vi "FOCUS_V42.vi"(9 "X-pixels":sgl=256.0, 11 "Run":bool) -> (0 "Retrace pixels":sgl, 10 "Pixel Clock (Hz)":sgl)   [LabVIEW 2010] (continued)
                      tunnel: w5383 -> [w5401 w5419]
                      tunnel: w5352 -> [w5400 w5418]
                      tunnel: [w5399 w5417] -> w5382
                      tunnel: [w5398 w5416] -> w5381
                      tunnel: [w5398 w5416] -> w5368
                      tunnel: w5367 -> [_ _]
                      tunnel: w5360 -> [w5397 _]
                      tunnel: w5359 -> [w5393 w5414]
                      tunnel: [w5395 w5412] -> w5341
                      tunnel: w5340 -> [w5394 _]
                      frame False {
                        n2972 = case shown="True" w5394 {
                          tunnel: [w5402 w5403] -> w5395
                          tunnel: w5393 -> [w5402 _]
                          frame False {
                          }
                          frame True {
                            n2973 = local read "scattering length [µm]"() -> (w5411:sgl)
                            n2974 = local read "z-step (um)"() -> (w5407:sgl)
                            n2975 = Divide(x=w5407, y=w5411) -> (x/y=w5408:sgl)
                            n2976 = Exponential(1:w5408) -> (0:w5409:sgl)
                            n2977 = local read "Intensity"() -> (w5410:sgl)
                            n2978 = local read "IntensityScaleMax"() -> (w5404:sgl)
                            n2979 = Multiply(x=w5410, y=w5409) -> (x*y=w5405:sgl)
                            n2980 = In Range and Coerce(upper limit=sgl 0.0, x=w5405, lower limit=w5404) -> (coerced(x)=w5403:sgl)  [unwired: 1 out]
                            n2981 = local write "Intensity"(w5403) -> ()
                          }
                        }
                        n2982 = Build Array(w5397, w5395) -> (w5396:dbl[])
                        n2983 = call-poly <vilib>:"DAQmx Write (Analog 1D DBL NChan 1Samp).vi"("task/channels in"=w5401, "data"=w5396, "error in"=w5400) -> ("task out"=w5398:refnum<k21>, "error out"=w5399:errorcluster)  [unwired: 10 in, 1 out]
                      }
                      frame True {
                        n2984 = local read "IntensityScaleMax"() -> (w5413:sgl)
                        n2985 = In Range and Coerce(upper limit=sgl 0.0, x=w5414, lower limit=w5413) -> (coerced(x)=w5412:sgl)  [unwired: 1 out]
                        n2986 = local write "Intensity"(w5412) -> ()
                        n2987 = Build Array(0.0 ("data"), w5412) -> (w5421:dbl[])
                        n2988 = call-poly <vilib>:"DAQmx Write (Analog 1D DBL NChan 1Samp).vi"("task/channels in"=w5419, "data"=w5421, "error in"=w5418) -> ("task out"=w5416:refnum<k21>, "error out"=w5417:errorcluster)  [unwired: 10 in, 1 out]
                      }
                    }
                    n2989 = case shown="False" w5326 {
                      tunnel: [w5431 w5457] -> w5371
                      tunnel: [w5430 w5456] -> w5370
                      tunnel: [w5428 w5454] -> w5356
                      tunnel: w5369 -> [w5427 w5457]
                      tunnel: w5368 -> [w5426 _]
                      tunnel: w5367 -> [w5425 w5456]
                      tunnel: w5358 -> [w5424 w5455]
                      tunnel: [w5423 w5455] -> w5357
                      tunnel: w5362 -> [w5422 w5454]
                      frame False {
                        n2990 = flat-sequence {
                          tunnel: sgl 100.0 ("Time interval [s]") -> [w5443]
                          tunnel: [w5443] -> w5437
                          tunnel: [w5439] -> w5436
                          tunnel: [w5438] -> w5435
                          tunnel: w5427 -> [w5441]
                          tunnel: w5425 -> [w5440]
                          tunnel: [w5450] -> w5434
                          tunnel: [w5449] -> w5433
                          tunnel: [w5448] -> w5432
                          tunnel: w5437 -> [w5450]
                          tunnel: w5436 -> [w5449]
                          tunnel: w5435 -> [w5448]
                          tunnel: w5424 -> [w5447]
                          tunnel: w5422 -> [w5446]
                          tunnel: [w5445] -> w5428
                          tunnel: [w5444] -> w5423
                          tunnel: [w5453] -> w5431
                          tunnel: w5434 -> [w5452]
                          tunnel: w5433 -> [w5453]
                          tunnel: w5432 -> [w5451]
                          tunnel: [w5451] -> w5430
                          tunnel: w5426 -> [_]
                          frame #0 {
                            w5442 = FALSE ("data")
                            n2991 = local write "Shutter open"(w5442) -> ()
                            n2992 = call-poly <vilib>:"DAQmx Write (Digital Bool 1Line 1Point).vi"("task/channels in"=w5441, "data"=w5442, "error in"=w5440) -> ("task out"=w5439:refnum<k21>, "error out"=w5438:errorcluster)  [unwired: 10 in, 1 out]
                          }
                          frame #1 {
                            n2993 = call <vilib>:"DAQmx Stop Task.vi"("task/channels in"=w5447, "error in"=w5446) -> ("task out"=w5444:refnum<k21>, "error out"=w5445:errorcluster)  [unwired: 12 in]
                          }
                          frame #2 {
                            n2994 = Wait (ms)(milliseconds to wait=w5452) -> ()  [unwired: 1 out]
                          }
                        }
                      }
                      frame True {
                      }
                    }
                    n2995 = call "ConvertImagesDataFOCUS.vi"("Save mode"=w5320, "Image3"=w5324, "Image2"=w5333, "Image1"=w5334) -> ("Data"=w5332:u8[])
                    n2996 = Set File Position(refnum=w5338, from (0:start)=enum16{"start", "end", "current"}."current" ("pos mode (0:2)"), error in=w5337) -> (refnum out=w5319:refnum<file>, error out=w5318:errorcluster)  [unwired: 1 in]
                    n2997 = Write to Binary File(file (use dialog)=w5319, data=w5332, error in=w5318, 5:FALSE ("prepend array or string size? (T)")) -> (refnum out=w5336:refnum<file>, error out=w5335:errorcluster)  [unwired: 2 in, 1 out]
                    n2998 = local read "Y-lines"() -> (w5380:sgl)
                    n2999 = Multiply(x=w5353, y=w5380) -> (x*y=w5378:sgl)
                    n3000 = Replace Array Subset(array=w5385, new element=w5334, index (row)=0 ("disabled index (row)"), index (col)=w5378) -> (w5384:u8[][])
                    n3001 = Replace Array Subset(array=w5387, new element=w5333, index (row)=0 ("disabled index (row)"), index (col)=w5378) -> (w5386:u8[][])
                  }
                  n3002 = Not Equal?(x=w5253, y=w5254) -> (x != y?=w5255:bool)
                  n3003 = local write "IntDevUsed"(w5255) -> ()
                  n3004 = Close File(refnum=w5240, error in=w5239) -> ()  [unwired: 2 out]
                  n3005 = flat-sequence {
                    tunnel: [w5302] -> w5264
                    tunnel: w5266 -> [w5302]
                    tunnel: w5265 -> [w5301]
                    tunnel: [w5301] -> w5263
                    frame #0 {
                      n3006 = Tick Count (ms)() -> (millisecond timer value=w5303:u32)
                      n3007 = local write "stop"(w5303) -> ()
                    }
                  }
                }
                frame 5 {
                  w5744 = sgl 1000000.0 ("y")
                  w5776 = 0.0 ("X Scale.Range:Minimum")
                  w5783 = TRUE ("Visible")
                  # "User-defined line 3D"
                  n3008 = Greater Or Equal?(x=w5710, y=u16 3) -> (x >= y?=w5708:bool)
                  n3009 = property on="Property Node" class="VI"() -> ("VI Path"=w5738:path)  [unwired: 2 in, 2 out]
                  n3010 = property on="Property Node" class="VI"() -> ("VI Path"=w5719:path)  [unwired: 2 in, 2 out]
                  n3011 = flat-sequence {
                    tunnel: w5785 -> [w5800]
                    tunnel: [w5800] -> w5784
                    frame #0 {
                      n3012 = Tick Count (ms)() -> (millisecond timer value=w5801:u32)
                      n3013 = local write "start"(w5801) -> ()
                    }
                  }
                  n3014 = Unbundle By Name(w5723) -> ("status"=w5757:bool)
                  n3015 = Increment(x=w5734) -> (x+1=w5733:sgl)
                  n3016 = Tick Count (ms)() -> (millisecond timer value=w5789:u32)
                  n3017 = Strip Path(path=w5738) -> (stripped path=w5737:path)  [unwired: 1 out]
                  n3018 = Strip Path(path=w5719) -> (stripped path=w5718:path)  [unwired: 1 out]
                  n3019 = local read "X-pixels FreeLine"() -> (w5743:sgl)
                  n3020 = local read "Y-lines FreeLine"() -> (w5745:sgl)
                  n3021 = Build Path(base path=w5737, name or relative path="FreeLine.tmp") -> (appended path=w5736:path)
                  n3022 = Build Path(base path=w5718, name or relative path="EEG.tmp") -> (appended path=w5717:path)
                  n3023 = call <vilib>:"Open_Create_Replace File.vi"("advisory dialog? (display:T)"=FALSE, "function (open:0)"=T8."create or replace", "file path"=w5736) -> ("error out"=w5727:errorcluster, "refnum"=w5729:refnum<file>)  [unwired: 5 in, 2 out]
                  n3024 = Unbundle By Name(w5759) -> ("status"=w5758:bool)
                  n3025 = call <vilib>:"Open_Create_Replace File.vi"("advisory dialog? (display:T)"=FALSE, "function (open:0)"=T8."create or replace", "file path"=w5717) -> ("error out"=w5715:errorcluster, "refnum"=w5714:refnum<file>)  [unwired: 5 in, 2 out]
                  n3026 = Divide(x=w5744, y=w5743) -> (x/y=w5742:sgl)
                  n3027 = Multiply(x=w5745, y=w5743) -> (x*y=w5746:sgl)
                  n3028 = local read "XScale"() -> (w5777:bool)
                  n3029 = Greater?(x=w5746, y=w5744) -> (0:w5747:bool)
                  n3030 = Select(t=w5742, s=w5747, f=w5745) -> (s? t:f=w5741:sgl)
                  n3031 = case shown="True" w5777 {
                    tunnel: [w5796 w5797] -> w5775
                    tunnel: w5741 -> [w5796 _]
                    tunnel: w5743 -> [_ w5797]
                    frame False {
                    }
                    frame True {
                    }
                  }
                  n3032 = Set File Position(refnum=w5729, from (0:start)=enum16{"start", "end", "current"}."start" ("pos mode (rel. to end:1)"), error in=w5727) -> (refnum out=w5707:refnum<file>, error out=w5706:errorcluster)  [unwired: 1 in]
                  n3033 = Write to Binary File(file (use dialog)=w5707, data=w5730, error in=w5706, 5:FALSE ("prepend array or string size? (T)")) -> (refnum out=w5728:refnum<file>, error out=w5726:errorcluster)  [unwired: 2 in, 1 out]
                  n3034 = while {
                    tunnel: [w5841] -> w5790
                    tunnel: [w5839] -> w5787
                    tunnel: w5791 -> [w5870]
                    tunnel: w5784 -> [w5863]
                    shift-right: [w5846] -> w5751
                    shift-left: w5792 -> [w5902]
                    tunnel: w5748 -> [w5817]
                    shift-right: [w5848] -> w5752
                    shift-left: w5792 -> [w5901]
                    shift-right: [w5896] -> _
                    shift-left: w5789 -> [w5897]
                    tunnel: w5781 -> [w5873]
                    tunnel: w5780 -> [w5864]
                    tunnel: [w5872] -> w5778
                    tunnel: [w5871] -> w5779
                    shift-right: [w5876] -> w5732
                    shift-left: w5774 -> [w5878]
                    tunnel: w5764 -> [w5874]
                    tunnel: w5763 -> [w5862]
                    tunnel: [w5874] -> w5761
                    tunnel: [w5862] -> w5762
                    tunnel: [w5866] -> w5760
                    tunnel: w5758 -> [w5861]
                    tunnel: w5757 -> [w5857]
                    shift-right: [w5850] -> w5749
                    shift-left: w5728 -> [w5852]
                    shift-right: [w5849] -> w5750
                    shift-left: w5726 -> [w5851]
                    tunnel: w5733 -> [w5843]
                    tunnel: w5725 -> [w5837]
                    tunnel: w5723 -> [w5836]
                    tunnel: [w5835] -> w5724
                    tunnel: [w5834] -> w5722
                    shift-right: [w5826] -> w5713
                    shift-left: w5714 -> [w5828]
                    shift-right: [w5825] -> w5712
                    shift-left: w5715 -> [w5827]
                    tunnel: w5711 -> [w5823]
                    tunnel: w5710 -> [w5813]
                    tunnel: w5708 -> [w5808]
                    i -> [w5844]
                    stop <- w5853 stop-if-true
                    # "DIO Read reads one\nline of data at a time"
                    n3035 = Unbundle By Name(w5862) -> ("status"=w5860:bool)
                    n3036 = Unbundle By Name(w5864) -> ("status"=w5859:bool)
                    n3037 = Equal To 0?(x=w5844) -> (x = 0?=w5883:bool)
                    n3038 = Unbundle By Name(w5863) -> ("status"=w5858:bool)
                    n3039 = local read "End experiment"() -> (w5855:bool)
                    n3040 = local read "Y-lines FreeLine"() -> (w5865:sgl)
                    n3041 = case shown="False" w5883 {
                      tunnel: w5817 -> [w5962 w5965]
                      tunnel: [w5962 w5964] -> w5816
                      tunnel: w5823 -> [_ w5963]
                      tunnel: [sgl 0.0 w5963] -> w5818
                      frame False {
                      }
                      frame True {
                        n3042 = Add(x=w5965, y=w5963) -> (x+y=w5964:sgl)
                      }
                    }
                    n3043 = call-poly <vilib>:"DAQmx Read (Analog 2D DBL NChan NSamp).vi"("task/channels in"=w5873, "number of samples per channel"=w5816, "error in"=w5864) -> ("task out"=w5872:refnum<k21>, "data"=w5820:dbl[][], "error out"=w5871:errorcluster)  [unwired: 10 in]
                    n3044 = Array Subset(array=w5820, index (col)=w5818) -> (w5819:dbl[][])  [unwired: 3 in]
                    n3045 = local read "stop 2"() -> (w5856:bool)
                    n3046 = Transpose 2D Array(2D array=w5819) -> (transposed array=w5830:dbl[][])
                    n3047 = Increment(x=w5844) -> (x+1=w5875:i32)
                    n3048 = call-poly <vilib>:"DAQmx Read (Digital 1D U32 1Chan NSamp).vi"("task/channels in"=w5870, "number of samples per channel"=w5816, "error in"=w5863) -> ("task out"=w5842:refnum<k21>, "data"=w5822:u32[], "error out"=w5840:errorcluster)  [unwired: 10 in]
                    n3049 = Build Array (concatenate)(w5878, w5830) -> (w5877:dbl[][])
                    n3050 = Multiply(x="z frequency", y=w5817) -> (x*y=w5833:dbl)
                    n3051 = Index Array(array=w5830, index (col)=0 ("disabled index (col)")) -> (element=w5880:dbl[])  [unwired: 1 in]
                    n3052 = Equal?(x=w5875, y=w5865) -> (x = y?=w5854:bool)
                    n3053 = local write "#"(w5875) -> ()
                    n3054 = Index Array(array=w5830, index (col)=1 ("disabled index (col)")) -> (element=w5879:dbl[])  [unwired: 1 in]
                    n3055 = Array Subset "Extract DI0"(array=w5822, index=w5818) -> (w5821:u32[])  [unwired: 1 in]
                    n3056 = Index Array(array=w5830, index (col)=3 ("disabled index (col)")) -> (element=w5824:dbl[])  [unwired: 1 in]
                    n3057 = local read "Overlay Images"() -> (w5884:bool)
                    n3058 = property class="DAQmx Timing"(reference=w5837, error in=w5836, "Sample Clock:Rate"=w5833) -> (reference out=w5835:refnum<k21>, error out=w5834:errorcluster)
                    n3059 = Compound Arithmetic op=OR(w5854, w5855, w5856, w5857, w5858, w5859, w5860, w5861) -> (w5853:bool)
                    n3060 = Array Subset(array=w5877, index (row)=w5817) -> (w5876:dbl[][])  [unwired: 3 in]
                    n3061 = local read "x scale"() -> (w5890:dbl)
                    n3062 = local read "y scale"() -> (w5888:dbl)
                    n3063 = Split Number(x=w5821) -> (hi(x)=w5815:u16[], lo(x)=w5814:u16[])
                    n3064 = property class="DAQmx Read"(reference=w5842, error in=w5840) -> (reference out=w5841:refnum<k21>, error out=w5839:errorcluster, "Status:Available Samples Per Channel"=→"Scan Backlock":u32)
                    n3065 = case shown="0, Default" w5813 {
                      tunnel: w5815 -> [w5914 w5919 w5924 w5929 w5934 w5939]
                      tunnel: [w5913 w5918 w5921 w5928 w5933 w5936] -> w5812
                      tunnel: [w5911 w5916 w5923 w5926 w5931 w5938] -> w5811
                      tunnel: w5814 -> [w5912 w5917 w5922 w5927 w5932 w5937]
                      tunnel: [w5910 w5915 w5920 w5925 w5930 w5935] -> w5810
                      frame 0, Default {
                        n3066 = Split Number(x=w5914) -> (hi(x)=w5913:u8[], lo(x)=w5911:u8[])
                        n3067 = Split Number(x=w5912) -> (lo(x)=w5910:u8[])  [unwired: 1 out]
                      }
                      frame 1 {
                        n3068 = Split Number(x=w5919) -> (hi(x)=w5918:u8[], lo(x)=w5915:u8[])
                        n3069 = Split Number(x=w5917) -> (lo(x)=w5916:u8[])  [unwired: 1 out]
                      }
                      frame 2 {
                        n3070 = Split Number(x=w5924) -> (hi(x)=w5920:u8[], lo(x)=w5923:u8[])
                        n3071 = Split Number(x=w5922) -> (lo(x)=w5921:u8[])  [unwired: 1 out]
                      }
                      frame 3 {
                        n3072 = Split Number(x=w5929) -> (hi(x)=w5928:u8[], lo(x)=w5926:u8[])
                        n3073 = Split Number(x=w5927) -> (lo(x)=w5925:u8[])  [unwired: 1 out]
                      }
                      frame 4 {
                        n3074 = Split Number(x=w5934) -> (hi(x)=w5933:u8[], lo(x)=w5930:u8[])
                        n3075 = Split Number(x=w5932) -> (lo(x)=w5931:u8[])  [unwired: 1 out]
                      }
                      frame 5 {
                        n3076 = Split Number(x=w5939) -> (hi(x)=w5935:u8[], lo(x)=w5938:u8[])
                        n3077 = Split Number(x=w5937) -> (lo(x)=w5936:u8[])  [unwired: 1 out]
                      }
                    }
                    n3078 = Tick Count (ms)() -> (millisecond timer value=w5898:u32)
                    n3079 = Multiply(x=w5879, y=w5888) -> (x*y=w5892:dbl[])
                    n3080 = Multiply(x=w5890, y=w5880) -> (x*y=w5894:dbl[])
                    n3081 = local read "x offset"() -> (w5889:dbl)
                    n3082 = case shown="True" w5884 {
                      tunnel: w5812 -> [w5967 w5970]
                      tunnel: [w5967 w5968] -> w5886
                      tunnel: w5811 -> [w5966 w5969]
                      tunnel: [w5966 _] -> w5885
                      frame False {
                      }
                      frame True {
                        n3083 = To Word Integer(number=w5970) -> (16bit integer=w5975:i16[])
                        n3084 = Subtract(x=w5975, y=w5969) -> (x-y=w5976:i16[])
                        n3085 = Add(x=w5975, y=w5969) -> (x+y=w5980:i16[])
                        n3086 = Increment(x=w5980) -> (x+1=w5971:i16[])
                        n3087 = Divide(x=w5976, y=w5971) -> (x/y=w5972:dbl[])
                        n3088 = Absolute Value(x=w5976) -> (abs(x)=w5978:i16[])
                        n3089 = Multiply(x=w5972, y=u8 2) -> (x*y=w5974:dbl[])
                        n3090 = Round To Nearest(number=w5974) -> (nearest integer value=w5987:dbl[])
                        n3091 = Divide(x=w5978, y=2.0) -> (x/y=w5981:dbl[])
                        n3092 = Divide(x=w5980, y=2.0) -> (x/y=w5982:dbl[])
                        n3093 = Add(x=w5981, y=w5982) -> (x+y=w5984:dbl[])
                        n3094 = Divide(x=w5984, y=5.0) -> (x/y=w5985:dbl[])
                        n3095 = Round To Nearest(number=w5985) -> (nearest integer value=w5986:dbl[])
                        n3096 = Multiply(x=5.0 ("y"), y=w5986) -> (x*y=w5988:dbl[])
                        n3097 = Add(x=w5987, y=w5988) -> (x+y=w5989:dbl[])
                        n3098 = Subtract(x=w5989, y=2.0) -> (x-y=w5992:dbl[])
                        n3099 = To Unsigned Byte Integer(number=w5992) -> (unsigned 8bit integer=w5968:u8[])
                      }
                    }
                    n3100 = Subtract(x=w5898, y=w5897) -> (x-y=w5899:u32)
                    n3101 = local read "y offset"() -> (w5887:dbl)
                    n3102 = local read "Image Update [ms]"() -> (w5869:u32)
                    n3103 = Add(x=w5892, y=w5887) -> (x+y=w5891:dbl[])
                    n3104 = Add(x=w5889, y=w5894) -> (x+y=w5893:dbl[])
                    n3105 = Subtract(x=w5844, y=w5817) -> (x-y=w5866:sgl)
                    n3106 = case shown="True" w5808 {
                      tunnel: w5812 -> [w5906 w5909]
                      tunnel: w5811 -> [w5903 w5908]
                      tunnel: w5810 -> [w5905 _]
                      tunnel: [w5904 w5907] -> w5809
                      frame True {
                        n3107 = Interleave 1D Arrays(w5903, w5906, w5905) -> (w5904:u8[])
                      }
                      frame False {
                        n3108 = Interleave 1D Arrays(w5909, w5908) -> (w5907:u8[])
                      }
                    }
                    n3109 = Multiply(x=w5869, y=u32 20) -> (x*y=w5867:u32)
                    n3110 = Greater Or Equal?(x=w5899, y=w5867) -> (x >= y?=w5900:bool)
                    n3111 = Greater Or Equal?(x=w5844, y=w5843) -> (x >= y?=w5845:bool)
                    n3112 = case shown="True" w5845 {
                      tunnel: w5902 -> [w5946 w5959]
                      tunnel: w5901 -> [w5945 w5953]
                      tunnel: w5886 -> [w5944 w5957]
                      tunnel: w5885 -> [w5943 w5950]
                      tunnel: [w5942 w5947] -> w5848
                      tunnel: [w5941 w5960] -> w5846
                      tunnel: w5844 -> [w5940 _]
                      frame False {
                        n3113 = Replace Array Subset(array=w5946, new element=w5944, index (col)=w5940) -> (w5941:u8[][])  [unwired: 1 in]
                        n3114 = Replace Array Subset(array=w5945, new element=w5943, index (col)=w5940) -> (w5942:u8[][])  [unwired: 1 in]
                      }
                      frame True {
                        n3115 = Transpose 2D Array(2D array=w5953) -> (transposed array=w5951:u8[][])
                        n3116 = Transpose 2D Array(2D array=w5959) -> (transposed array=w5958:u8[][])
                        n3117 = Build Array (concatenate)(w5951, w5950) -> (w5952:u8[][])
                        n3118 = Build Array (concatenate)(w5958, w5957) -> (w5956:u8[][])
                        n3119 = Transpose 2D Array(2D array=w5952) -> (transposed array=w5948:u8[][])
                        n3120 = Transpose 2D Array(2D array=w5956) -> (transposed array=w5955:u8[][])
                        n3121 = Array Subset(array=w5955, index (col)=1 ("index")) -> (w5960:u8[][])  [unwired: 3 in]
                        n3122 = Array Subset(array=w5948, index (col)=1 ("index")) -> (w5947:u8[][])  [unwired: 3 in]
                      }
                    }
                    n3123 = Set File Position(refnum=w5828, from (0:start)=enum16{"start", "end", "current"}."current" ("pos mode (0:2)"), error in=w5827) -> (refnum out=w5807:refnum<file>, error out=w5806:errorcluster)  [unwired: 1 in]
                    n3124 = Write to Binary File(file (use dialog)=w5807, data=w5824, error in=w5806, 5:FALSE ("prepend array or string size? (T)")) -> (refnum out=w5826:refnum<file>, error out=w5825:errorcluster)  [unwired: 2 in, 1 out]
                    n3125 = Set File Position(refnum=w5852, from (0:start)=enum16{"start", "end", "current"}."current" ("pos mode (0:2)"), error in=w5851) -> (refnum out=w5804:refnum<file>, error out=w5803:errorcluster)  [unwired: 1 in]
                    n3126 = Write to Binary File(file (use dialog)=w5804, data=w5809, error in=w5803, 5:FALSE ("prepend array or string size? (T)")) -> (refnum out=w5850:refnum<file>, error out=w5849:errorcluster)  [unwired: 2 in, 1 out]
                    n3127 = Bundle(w5893, w5891) -> (w5895:cluster{dbl[], dbl[]})  [unwired: 1 in]
                    n3128 = case shown="True" w5900 {
                      tunnel: [w5993 w5997] -> w5896
                      tunnel: w5897 -> [w5993 _]
                      tunnel: w5895 -> [_ w5996]
                      tunnel: w5846 -> [_ w5995]
                      tunnel: w5848 -> [_ w5994]
                      frame False {
                      }
                      frame True {
                        n3129 = local write "XY Graph 3"(w5996) -> ()
                        n3130 = local write "XY Graph 4"(w5996) -> ()
                        n3131 = local write "Image 4"(w5994) -> ()
                        n3132 = local write "Image 3"(w5995) -> ()
                        n3133 = Tick Count (ms)() -> (millisecond timer value=w5997:u32)
                      }
                    }
                  }
                  n3134 = property on="Image 2" class="IntGraph (strict)"() -> ("Color Table"=w5782:u32[])  [unwired: 2 in, 2 out]
                  n3135 = property on="Image 3" class="IntGraph (strict)"("X Scale.Range:Minimum"=w5776, "X Scale.Range:Maximum"=w5775, "Y Scale.Range:Minimum"=w5776, "Y Scale.Range:Maximum"=w5741, "Visible"=w5783, "Color Table"=w5782) -> ()  [unwired: 2 in, 2 out]
                  n3136 = property on="Image 4" class="IntGraph (strict)"("X Scale.Range:Minimum"=w5776, "X Scale.Range:Maximum"=w5775, "Y Scale.Range:Minimum"=w5776, "Y Scale.Range:Maximum"=w5741, "Visible"=w5783, "Color Table"=w5782) -> ()  [unwired: 2 in, 2 out]
                  n3137 = property on="Histogram1" class="XYGraph (strict)"("X Scale.Range:Minimum"=w5776, "X Scale.Range:Maximum"=w5775) -> ()  [unwired: 2 in, 2 out]
                  n3138 = property on="Histogram2" class="XYGraph (strict)"("X Scale.Range:Minimum"=w5776, "X Scale.Range:Maximum"=w5775) -> ()  [unwired: 2 in, 2 out]
                  n3139 = Close File(refnum=w5749, error in=w5750) -> ()  [unwired: 2 out]
                  n3140 = Close File(refnum=w5713, error in=w5712) -> ()  [unwired: 2 out]
                  n3141 = Array Subset(array=w5732, index (col)=0 ("index"), length (col)=3 ("length")) -> (w5765:dbl[][])  [unwired: 2 in]
                  n3142 = Index Array(array=w5765, index (col)=0 ("disabled index (col)")) -> (element=w5772:dbl[])  [unwired: 1 in]
                  n3143 = flat-sequence {
                    tunnel: w5787 -> [w5798]
                    tunnel: [w5798] -> w5786
                    frame #0 {
                      n3144 = Tick Count (ms)() -> (millisecond timer value=w5799:u32)
                      n3145 = local write "stop"(w5799) -> ()
                    }
                  }
                  n3146 = Array Size(array=w5772) -> (size(s)=w5771:i32)
                  n3147 = Multiply(x=w5771, y=3) -> (x*y=w5769:i32)
                  n3148 = Reshape Array(w5765, w5769) -> (w5768:dbl[])
                  n3149 = local write "Positions"(w5768) -> ()
                }
              }
            }
            frame True {
              n3150 = local read "scans to read"() -> (w6007:sgl)
              n3151 = local read "Number of Frames"() -> (w6004:sgl)
              n3152 = Multiply(x=w6007, y=w6006) -> (x*y=w6003:sgl)
              n3153 = Multiply(x=w6005, y=w6004) -> (x*y=w6010:sgl)
              n3154 = Reciprocal(x=w6003) -> (1/x=w6002:sgl)
              n3155 = local write "Frame rate [Hz]"(w6002) -> ()
              n3156 = case shown="0, Default" w6050 {
                tunnel: w6049 -> [w6084 w6319 w6507]
                tunnel: w6048 -> [w6085 w6320 w6508]
                tunnel: w6047 -> [w6073 w6308 w6496]
                tunnel: w6046 -> [w6083 w6318 w6506]
                tunnel: w6045 -> [w6072 w6307 w6495]
                tunnel: w6044 -> [w6078 w6313 w6501]
                tunnel: w6043 -> [w6077 w6312 w6500]
                tunnel: w6042 -> [w6082 w6317 w6505]
                tunnel: w6041 -> [w6081 w6316 w6504]
                tunnel: w6040 -> [w6087 w6298 w6486]
                tunnel: w6039 -> [w6068 w6297 w6485]
                tunnel: w6038 -> [w6088 w6322 w6510]
                tunnel: w6037 -> [w6069 w6304 w6492]
                tunnel: w6036 -> [w6089 w6323 w6511]
                tunnel: [w6089 w6323 w6511] -> w6035
                tunnel: [w6069 w6304 w6492] -> w6033
                tunnel: [w6088 w6322 w6510] -> w6034
                tunnel: [w6068 w6295 w6483] -> w6031
                tunnel: [w6087 w6296 w6484] -> w6032
                tunnel: [768 ("DataOffset") 768 ("DataOffset") 768 ("DataOffset")] -> w6030
                tunnel: [0 ("DataOffset") 0 ("DataOffset") 0 ("DataOffset")] -> w6029
                tunnel: [0 ("DataOffset") 0 ("DataOffset") 0 ("DataOffset")] -> w6028
                tunnel: [w6079 w6314 w6502] -> w6027
                tunnel: [w6080 w6315 w6503] -> w6026
                tunnel: [w6075 w6310 w6498] -> w6025
                tunnel: [w6076 w6311 w6499] -> w6024
                tunnel: [w6073 w6308 w6496] -> w6023
                tunnel: [w6085 w6320 w6508] -> w6022
                tunnel: [w6084 w6319 w6507] -> w6021
                tunnel: [w6072 w6307 w6495] -> w6020
                tunnel: [w6083 w6318 w6506] -> w6019
                tunnel: w6018 -> [w6055 w6283 w6497]
                tunnel: w6017 -> [w6062 w6301 w6489]
                tunnel: w6007 -> [_ w6290 w6482]
                tunnel: w6016 -> [w6061 w6289 w6481]
                tunnel: w6015 -> [w6060 w6288 w6480]
                tunnel: w6014 -> [w6059 w6286 w6478]
                tunnel: w6013 -> [w6058 w6287 w6479]
                tunnel: [w6057 w6286 w6478] -> w6012
                tunnel: [w6056 w6287 w6479] -> w6011
                tunnel: w6010 -> [_ w6285 _]
                tunnel: w6009 -> [_ w6284 _]
                tunnel: [_ w6281 w6473] -> w6008
                tunnel: w6006 -> [w6053 _ _]
                tunnel: [w6052 w6279 w6472] -> w6001
                tunnel: [w6051 w6278 w6471] -> w6000
                frame 0, Default {
                  # "Focus mode FScope"
                  n3157 = To Unsigned Long Integer(number=w6055) -> (unsigned 32bit integer=w6054:u32[][])
                  n3158 = Tick Count (ms)() -> (millisecond timer value=w6074:u32)
                  n3159 = Unbundle By Name(w6073) -> ("status"=w6071:bool)
                  n3160 = Unbundle By Name(w6072) -> ("status"=w6070:bool)
                  n3161 = Unbundle By Name(w6068) -> ("status"=w6067:bool)
                  n3162 = Unbundle By Name(w6069) -> ("status"=w6066:bool)
                  n3163 = while {
                    tunnel: w6082 -> [w6167]
                    tunnel: w6081 -> [w6166]
                    tunnel: [w6165] -> w6080
                    tunnel: [w6154] -> w6079
                    shift-right: [w6144] -> w6052
                    shift-left: w6055 -> [w6134]
                    shift-right: [w6115] -> w6051
                    shift-left: w6055 -> [w6131]
                    tunnel: [w6159] -> w6076
                    tunnel: w6078 -> [w6159]
                    tunnel: [w6155] -> w6075
                    tunnel: w6077 -> [w6155]
                    shift-right: [w6142] -> _
                    shift-left: w6074 -> [w6143]
                    shift-right: [w6097] -> _
                    shift-left: w6054 -> [w6137]
                    tunnel: w6071 -> [w6151]
                    tunnel: w6070 -> [w6156]
                    tunnel: w6067 -> [w6150]
                    tunnel: w6066 -> [w6149]
                    shift-right: [w6140] -> _
                    shift-left: 0.0 ("millisecond timer value") -> [w6119]
                    tunnel: w6062 -> [w6139]
                    shift-right: [w6122] -> _
                    shift-left: w6060 -> [w6124]
                    shift-right: [w6121] -> _
                    shift-left: w6061 -> [w6123]
                    tunnel: w6059 -> [w6103]
                    tunnel: w6058 -> [w6102]
                    tunnel: [w6101] -> w6057
                    tunnel: [w6100] -> w6056
                    tunnel: w6053 -> [w6093]
                    stop <- w6148 stop-if-true
                    n3164 = Multiply(x="scans to read", y=w6093) -> (x*y=w6091:sgl)
                    n3165 = Bundle("ScaleCluster"="ScaleCluster", "scans to read"="scans to read") -> (w6122:T20)  [unwired: 1 in]
                    n3166 = Reciprocal(x=w6091) -> (1/x=→"Frame rate [Hz]":sgl)
                    n3167 = call-poly <vilib>:"DAQmx Read (Digital 1D U32 1Chan NSamp).vi"("task/channels in"=w6167, "number of samples per channel"="scans to read", "error in"=w6166) -> ("task out"=w6165:refnum<k21>, "data"=w6095:u32[], "error out"=w6154:errorcluster)  [unwired: 10 in]
                    n3168 = local read "Overlay Images"() -> (w6162:bool)
                    n3169 = Not Equal?(x=w6122, y=w6124) -> (x != y?=w6125:bool)
                    n3170 = Multiply(x=u32 0 ("millisecond timer value"), y=w6137) -> (x*y=w6136:u32[][])
                    n3171 = case shown="True" w6125 {
                      tunnel: w6139 -> [_ w6246]
                      tunnel: w6122 -> [_ w6245]
                      tunnel: [w6243 w6244] -> w6121
                      tunnel: w6123 -> [w6243 _]
                      frame False {
                      }
                      frame True {
                        n3172 = call "ScaleScanlineFScope.vi"("Parameters"=w6246, "ScaleCluster"=w6245) -> ("ScanlineScaled"=w6244:dbl[][])
                      }
                    }
                    n3173 = Split Number(x=w6095) -> (hi(x)=w6164:u16[])  [unwired: 1 out]
                    n3174 = Multiply(x=u8 0 ("millisecond timer value"), y=w6134) -> (x*y=w6133:u8[][])
                    n3175 = Split Number(x=w6164) -> (hi(x)=w6110:u8[], lo(x)=w6163:u8[])
                    n3176 = call-poly <vilib>:"Ramp Pattern.vi"("start"=0.0, "end"=6.283185307179586, "samples"="scans to read") -> ("Ramp Pattern"=w6114:dbl[])  [unwired: 7 in, 1 out]
                    n3177 = case shown="True" w6162 {
                      tunnel: w6110 -> [w6252 w6271]
                      tunnel: [w6252 w6254] -> w6146
                      tunnel: w6163 -> [w6251 w6273]
                      tunnel: [w6251 _] -> w6145
                      frame False {
                      }
                      frame True {
                        n3178 = To Word Integer(number=w6271) -> (16bit integer=w6272:i16[])
                        n3179 = Subtract(x=w6272, y=w6273) -> (x-y=w6253:i16[])
                        n3180 = Add(x=w6272, y=w6273) -> (x+y=w6267:i16[])
                        n3181 = Increment(x=w6267) -> (x+1=w6277:i16[])
                        n3182 = Divide(x=w6253, y=w6277) -> (x/y=w6276:dbl[])
                        n3183 = Absolute Value(x=w6253) -> (abs(x)=w6269:i16[])
                        n3184 = Multiply(x=w6276, y=u8 2) -> (x*y=w6274:dbl[])
                        n3185 = Round To Nearest(number=w6274) -> (nearest integer value=w6260:dbl[])
                        n3186 = Divide(x=w6269, y=2.0) -> (x/y=w6266:dbl[])
                        n3187 = Divide(x=w6267, y=2.0) -> (x/y=w6265:dbl[])
                        n3188 = Add(x=w6266, y=w6265) -> (x+y=w6263:dbl[])
                        n3189 = Divide(x=w6263, y=5.0) -> (x/y=w6262:dbl[])
                        n3190 = Round To Nearest(number=w6262) -> (nearest integer value=w6261:dbl[])
                        n3191 = Multiply(x=5.0 ("y"), y=w6261) -> (x*y=w6259:dbl[])
                        n3192 = Add(x=w6260, y=w6259) -> (x+y=w6258:dbl[])
                        n3193 = Subtract(x=w6258, y=2.0) -> (x-y=w6255:dbl[])
                        n3194 = To Unsigned Byte Integer(number=w6255) -> (unsigned 8bit integer=w6254:u8[])
                      }
                    }
                    n3195 = Multiply(x=u8 0 ("millisecond timer value"), y=w6131) -> (x*y=w6130:u8[][])
                    n3196 = Sine(x=w6114) -> (sin(x)=w6112:dbl[])
                    n3197 = Array Subset(array=w6121, index (col)=w6119, length (col)="scans to read") -> (w6126:dbl[][])  [unwired: 2 in]
                    n3198 = Add(x=w6112, y=sgl 2.0 ("millisecond timer value")) -> (x+y=w6106:dbl[])
                    n3199 = Index Array(array=w6121, index (row)=0) -> (element=w6128:dbl[])  [unwired: 1 in]
                    n3200 = Divide(x=u32 4294967295 ("millisecond timer value"), y=sgl 3.0) -> (x/y=w6107:sgl)
                    n3201 = Array Size(array=w6128) -> (size(s)=w6117:i32)
                    n3202 = Multiply(x=w6107, y=w6106) -> (x*y=w6105:dbl[])
                    n3203 = Add(x=w6119, y="scans to read") -> (x+y=w6127:dbl)
                    n3204 = Divide(x=w6117, y=2) -> (x/y=w6116:dbl)
                    n3205 = To Unsigned Long Integer(number=w6105) -> ()  [unwired: 1 out]
                    n3206 = Greater Or Equal?(x=w6127, y=w6116) -> (x >= y?=w6141:bool)
                    n3207 = case shown="True" w6141 {
                      tunnel: w6127 -> [w6247 w6250]
                      tunnel: [w6247 w6248] -> w6140
                      tunnel: w6116 -> [_ w6249]
                      frame False {
                      }
                      frame True {
                        n3208 = Subtract(x=w6250, y=w6249) -> (x-y=w6248:dbl)
                      }
                    }
                    n3209 = Tick Count (ms)() -> (millisecond timer value=w6161:u32)
                    n3210 = local read "Image Update [ms]"() -> (w6158:u32)
                    n3211 = call "AverageImageFScope.vi"("HitsArray"=w6136, "ScanLineFScope"=w6126, "Image1Array"=w6133, "Image2Array"=w6130, "DataImage2"=w6145, "DataImage1"=w6146) -> ("HitsArraynew"=w6097:u32[][], "Image1Arraynew"=w6144:u8[][], "Image2Arraynew"=w6115:u8[][])
                    n3212 = Subtract(x=w6161, y=w6143) -> (x-y=w6160:u32)
                    n3213 = Greater Or Equal?(x=w6160, y=w6158) -> ()  [unwired: 1 out]
                    n3214 = local write "Image 1"(w6144) -> ()
                    n3215 = local write "Image 2"(w6115) -> ()
                    n3216 = local write "Hit Graph"(w6097) -> ()
                    n3217 = Unbundle By Name(w6155) -> ("status"=w6153:bool)
                    n3218 = Unbundle By Name(w6154) -> ("status"=w6152:bool)
                    n3219 = event shown="[1] \"Up 100\": Mouse Down" {
                      selector: _ -> [_ _ _ _ _ _ _]
                      dyn-events: _ -> [_ _ _ _ _ _ _]
                      timeout: 0 -> [_ _ _ _ _ _ _]
                      tunnel: w6103 -> [w6169 w6182 w6194 w6206 w6218 w6230 w6242]
                      tunnel: w6102 -> [w6168 w6181 w6193 w6205 w6217 w6229 w6241]
                      tunnel: [w6169 w6177 w6189 w6201 w6213 w6225 w6237] -> w6101
                      tunnel: [w6168 w6176 w6188 w6200 w6212 w6224 w6236] -> w6100
                      tunnel: [w6170 w6171 w6183 w6195 w6209 w6221 w6233] -> w6098
                      event Timeout {
                        n3220 = event-data() -> ()  [unwired: 1 in, 2 out]
                        n3221 = global read "GlobelFSCOPE.vi" "Focus"() -> (w6170:dbl)
                      }
                      event "Up 100": Mouse Down {
                        n3222 = event-data() -> ()  [unwired: 1 in, 1 out]
                        n3223 = Multiply(x=100.0 ("y"), y=0.3763) -> (x*y=w6173:dbl)
                        n3224 = call "MotorDriveFOCUS.vi"("task in"=w6182, "interdelay (ms)"=i16 3, "Iterations"=100, "error in"=w6181, "Up / Down"=TRUE) -> ("task out"=w6177:refnum<k21>, "error out"=w6176:errorcluster)
                        n3225 = global read "GlobelFSCOPE.vi" "Focus"() -> (w6172:dbl)
                        n3226 = Add(x=w6173, y=w6172) -> (x+y=w6171:dbl)
                        n3227 = global write "GlobelFSCOPE.vi" "Focus"(w6171) -> ()
                      }
                      event "Up 10": Mouse Down {
                        n3228 = event-data() -> ()  [unwired: 1 in, 1 out]
                        n3229 = Multiply(x=10.0 ("y"), y=0.3763) -> (x*y=w6186:dbl)
                        n3230 = call "MotorDriveFOCUS.vi"("task in"=w6194, "interdelay (ms)"=i16 3, "Iterations"=10, "error in"=w6193, "Up / Down"=TRUE) -> ("task out"=w6189:refnum<k21>, "error out"=w6188:errorcluster)
                        n3231 = global read "GlobelFSCOPE.vi" "Focus"() -> (w6185:dbl)
                        n3232 = Add(x=w6186, y=w6185) -> (x+y=w6183:dbl)
                        n3233 = global write "GlobelFSCOPE.vi" "Focus"(w6183) -> ()
                      }
                      event "Up 1": Mouse Down {
                        n3234 = event-data() -> ()  [unwired: 1 in, 1 out]
                        n3235 = Multiply(x=1.0 ("y"), y=0.3763) -> (x*y=w6198:dbl)
                        n3236 = call "MotorDriveFOCUS.vi"("task in"=w6206, "interdelay (ms)"=i16 3, "Iterations"=1, "error in"=w6205, "Up / Down"=TRUE) -> ("task out"=w6201:refnum<k21>, "error out"=w6200:errorcluster)
                        n3237 = global read "GlobelFSCOPE.vi" "Focus"() -> (w6199:dbl)
                        n3238 = Add(x=w6198, y=w6199) -> (x+y=w6195:dbl)
                        n3239 = global write "GlobelFSCOPE.vi" "Focus"(w6195) -> ()
                      }
                      event "Down 100": Mouse Down {
                        n3240 = event-data() -> ()  [unwired: 1 in, 1 out]
                        n3241 = Multiply(x=100.0 ("y"), y=0.3763) -> (x*y=w6207:dbl)
                        n3242 = call "MotorDriveFOCUS.vi"("task in"=w6218, "interdelay (ms)"=i16 3, "Iterations"=100, "error in"=w6217, "Up / Down"=FALSE) -> ("task out"=w6213:refnum<k21>, "error out"=w6212:errorcluster)
                        n3243 = global read "GlobelFSCOPE.vi" "Focus"() -> (w6208:dbl)
                        n3244 = Subtract(x=w6208, y=w6207) -> (x-y=w6209:dbl)
                        n3245 = global write "GlobelFSCOPE.vi" "Focus"(w6209) -> ()
                      }
                      event "Down 10": Mouse Down {
                        n3246 = event-data() -> ()  [unwired: 1 in, 1 out]
                        n3247 = Multiply(x=10.0 ("y"), y=0.3763) -> (x*y=w6219:dbl)
                        n3248 = call "MotorDriveFOCUS.vi"("task in"=w6230, "interdelay (ms)"=i16 3, "Iterations"=10, "error in"=w6229, "Up / Down"=FALSE) -> ("task out"=w6225:refnum<k21>, "error out"=w6224:errorcluster)
                        n3249 = global read "GlobelFSCOPE.vi" "Focus"() -> (w6220:dbl)
                        n3250 = Subtract(x=w6220, y=w6219) -> (x-y=w6221:dbl)
                        n3251 = global write "GlobelFSCOPE.vi" "Focus"(w6221) -> ()
                      }
                      event "Down 1": Mouse Down {
                        n3252 = event-data() -> ()  [unwired: 1 in, 1 out]
                        n3253 = Multiply(x=1.0 ("y"), y=0.3763) -> (x*y=w6232:dbl)
                        n3254 = call "MotorDriveFOCUS.vi"("task in"=w6242, "interdelay (ms)"=i16 3, "Iterations"=1, "error in"=w6241, "Up / Down"=FALSE) -> ("task out"=w6237:refnum<k21>, "error out"=w6236:errorcluster)
                        n3255 = global read "GlobelFSCOPE.vi" "Focus"() -> (w6231:dbl)
                        n3256 = Subtract(x=w6231, y=w6232) -> (x-y=w6233:dbl)
                        n3257 = global write "GlobelFSCOPE.vi" "Focus"(w6233) -> ()
                      }
                    }
                    n3258 = property on="Hit Graph" class="IntGraph (strict)"("Z Scale.Range:Minimum"=1.0, "Z Scale.Range:Maximum"="Scale") -> ()  [unwired: 2 in, 2 out]
                    n3259 = local read "stop 2"() -> (w6157:bool)
                    n3260 = local read "End experiment"() -> (w6147:bool)
                    n3261 = Tick Count (ms)() -> (millisecond timer value=w6142:u32)
                    n3262 = Compound Arithmetic op=OR(w6157, w6156, w6153, w6152, w6151, w6150, w6149, w6147) -> (w6148:bool)
                    n3263 = local write "Focus"(w6098) -> ()
                  }
                }
                frame 1 {
                  # "Frame scan FScope"
                  n3264 = Initialize Array(u8 0 ("element"), w6284, w6285) -> (w6291:u8[][])
                  n3265 = Tick Count (ms)() -> (millisecond timer value=w6309:u32)
                  n3266 = To Unsigned Long Integer(number=w6283) -> (unsigned 32bit integer=w6282:u32[][])
                  n3267 = Unbundle By Name(w6308) -> ("status"=w6306:bool)
                  n3268 = Unbundle By Name(w6307) -> ("status"=w6305:bool)
                  n3269 = Unbundle By Name(w6304) -> ("status"=w6303:bool)
                  n3270 = while {
                    tunnel: w6317 -> [w6407]
                    tunnel: w6316 -> [w6406]
                    tunnel: [w6405] -> w6315
                    tunnel: [w6394] -> w6314
                    shift-right: [w6368] -> _
                    shift-left: w6283 -> [w6363]
                    shift-right: [w6367] -> _
                    shift-left: w6283 -> [w6362]
                    tunnel: [w6399] -> w6311
                    tunnel: w6313 -> [w6399]
                    tunnel: [w6395] -> w6310
                    tunnel: w6312 -> [w6395]
                    shift-right: [w6385] -> _
                    shift-left: w6309 -> [w6386]
                    shift-right: [w6369] -> _
                    shift-left: w6282 -> [w6364]
                    tunnel: w6306 -> [w6391]
                    tunnel: w6305 -> [w6396]
                    tunnel: w6303 -> [w6371]
                    shift-right: [w6381] -> _
                    shift-left: sgl 0.0 ("millisecond timer value") -> [w6384]
                    tunnel: w6301 -> [w6380]
                    shift-right: [w6375] -> _
                    shift-left: sgl 1.0 ("millisecond timer value") -> [w6327]
                    tunnel: w6298 -> [w6378]
                    tunnel: [w6378] -> w6296
                    tunnel: [w6377] -> w6295
                    tunnel: w6297 -> [w6377]
                    shift-right: [w6365] -> _
                    shift-left: sgl 0.0 ("millisecond timer value") -> [w6366]
                    shift-right: [w6359] -> w6279
                    shift-left: w6291 -> [w6361]
                    shift-right: [w6358] -> w6278
                    shift-left: w6291 -> [w6360]
                    tunnel: w6290 -> [w6332]
                    shift-right: [w6348] -> _
                    shift-left: w6288 -> [w6350]
                    shift-right: [w6346] -> _
                    shift-left: w6289 -> [w6347]
                    tunnel: [w6325] -> w6280
                    i -> [w6330]
                    stop <- w6390 stop-if-true
                    n3271 = local read "ScaleCluster"() -> (w6357:T3)
                    n3272 = local read "Overlay Images"() -> (w6402:bool)
                    n3273 = Bundle("ScaleCluster"=w6357, "scans to read"=w6332) -> (w6348:T20)  [unwired: 1 in]
                    n3274 = call-poly <vilib>:"DAQmx Read (Digital 1D U32 1Chan NSamp).vi"("task/channels in"=w6407, "number of samples per channel"=w6332, "error in"=w6406) -> ("task out"=w6405:refnum<k21>, "data"=w6324:u32[], "error out"=w6394:errorcluster)  [unwired: 10 in]
                    n3275 = Not Equal?(x=w6348, y=w6350) -> (x != y?=w6349:bool)
                    n3276 = call-poly <vilib>:"Ramp Pattern.vi"("start"=0.0, "end"=6.283185307179586, "samples"=w6332) -> ("Ramp Pattern"=w6341:dbl[])  [unwired: 7 in, 1 out]
                    n3277 = case shown="True" w6349 {
                      tunnel: w6380 -> [_ w6411]
                      tunnel: [w6408 w6410] -> w6346
                      tunnel: w6348 -> [_ w6409]
                      tunnel: w6347 -> [w6408 _]
                      frame False {
                      }
                      frame True {
                        n3278 = call "ScaleScanlineFScope.vi"("Parameters"=w6411, "ScaleCluster"=w6409) -> ("ScanlineScaled"=w6410:dbl[][])
                      }
                    }
                    n3279 = Split Number(x=w6324) -> (hi(x)=w6404:u16[])  [unwired: 1 out]
                    n3280 = Sine(x=w6341) -> (sin(x)=w6339:dbl[])
                    n3281 = Split Number(x=w6404) -> (hi(x)=w6342:u8[], lo(x)=w6403:u8[])
                    n3282 = case shown="False" w6402 {
                      tunnel: w6342 -> [w6445 w6464]
                      tunnel: [w6445 w6447] -> w6388
                      tunnel: w6403 -> [w6444 w6466]
                      tunnel: [w6444 _] -> w6387
                      frame False {
                      }
                      frame True {
                        n3283 = To Word Integer(number=w6464) -> (16bit integer=w6465:i16[])
                        n3284 = Subtract(x=w6465, y=w6466) -> (x-y=w6446:i16[])
                        n3285 = Add(x=w6465, y=w6466) -> (x+y=w6460:i16[])
                        n3286 = Increment(x=w6460) -> (x+1=w6470:i16[])
                        n3287 = Divide(x=w6446, y=w6470) -> (x/y=w6469:dbl[])
                        n3288 = Absolute Value(x=w6446) -> (abs(x)=w6462:i16[])
                        n3289 = Multiply(x=w6469, y=u8 2) -> (x*y=w6467:dbl[])
                        n3290 = Round To Nearest(number=w6467) -> (nearest integer value=w6453:dbl[])
                        n3291 = Divide(x=w6462, y=2.0) -> (x/y=w6459:dbl[])
                        n3292 = Divide(x=w6460, y=2.0) -> (x/y=w6458:dbl[])
                        n3293 = Add(x=w6459, y=w6458) -> (x+y=w6456:dbl[])
                        n3294 = Divide(x=w6456, y=5.0) -> (x/y=w6455:dbl[])
                        n3295 = Round To Nearest(number=w6455) -> (nearest integer value=w6454:dbl[])
                        n3296 = Multiply(x=5.0 ("y"), y=w6454) -> (x*y=w6452:dbl[])
                        n3297 = Add(x=w6453, y=w6452) -> (x+y=w6451:dbl[])
                        n3298 = Subtract(x=w6451, y=2.0) -> (x-y=w6448:dbl[])
                        n3299 = To Unsigned Byte Integer(number=w6448) -> (unsigned 8bit integer=w6447:u8[])
                      }
                    }
                    n3300 = Add(x=w6339, y=sgl 2.0 ("millisecond timer value")) -> (x+y=w6334:dbl[])
                    n3301 = Divide(x=u32 4294967295 ("millisecond timer value"), y=sgl 3.0) -> (x/y=w6335:sgl)
                    n3302 = Array Subset(array=w6346, index (col)=w6384, length (col)=w6332) -> (w6354:dbl[][])  [unwired: 2 in]
                    n3303 = Multiply(x=w6335, y=w6334) -> (x*y=w6333:dbl[])
                    n3304 = To Unsigned Long Integer(number=w6333) -> ()  [unwired: 1 out]
                    n3305 = Index Array(array=w6346, index (row)=0) -> (element=w6355:dbl[])  [unwired: 1 in]
                    n3306 = Array Size(array=w6355) -> (size(s)=w6352:i32)
                    n3307 = Divide(x=w6352, y=2) -> (x/y=w6351:dbl)
                    n3308 = Add(x=w6384, y=w6332) -> (x+y=w6382:dbl)
                    n3309 = Greater Or Equal?(x=w6382, y=w6351) -> (x >= y?=w6383:bool)
                    n3310 = case shown="True" w6383 {
                      tunnel: w6382 -> [w6440 w6443]
                      tunnel: [w6440 w6441] -> w6381
                      tunnel: w6351 -> [_ w6442]
                      frame False {
                      }
                      frame True {
                        n3311 = Subtract(x=w6443, y=w6442) -> (x-y=w6441:dbl)
                      }
                    }
                    n3312 = Multiply(x="Averaging", y="Number of Frames") -> (x*y=w6373:sgl)
                    n3313 = Tick Count (ms)() -> (millisecond timer value=w6401:u32)
                    n3314 = Decrement(x=w6373) -> (x-1=w6372:sgl)
                    n3315 = Equal?(x="Averaging", y=w6327) -> (x = y?=w6376:bool)
                    n3316 = local read "Image Update [ms]"() -> (w6398:u32)
                    n3317 = Equal?(x=w6372, y=w6330) -> (x = y?=w6370:bool)
                    n3318 = call "AverageImageFScope.vi"("HitsArray"=w6364, "ScanLineFScope"=w6354, "Image1Array"=w6363, "Image2Array"=w6362, "DataImage2"=w6387, "DataImage1"=w6388) -> ("HitsArraynew"=w6345:u32[][], "Image1Arraynew"=w6344:u8[][], "Image2Arraynew"=w6343:u8[][])
                    n3319 = Subtract(x=w6401, y=w6386) -> (x-y=w6400:u32)
                    n3320 = Increment(x=w6330) -> (x+1=w6329:i32)
                    n3321 = Greater Or Equal?(x=w6400, y=w6398) -> ()  [unwired: 1 out]
                    n3322 = Divide(x=w6329, y="Averaging") -> (x/y=w6326:sgl)
                    n3323 = local write "Hit Graph"(w6345) -> ()
                    n3324 = local write "Image 1"(w6344) -> ()
                    n3325 = local write "Image 2"(w6343) -> ()
                    n3326 = case shown="True" w6376 {
                      tunnel: w6343 -> [w6419 w6423]
                      tunnel: w6344 -> [w6418 w6428]
                      tunnel: w6345 -> [w6417 w6436]
                      tunnel: [w6417 w6435] -> w6369
                      tunnel: [w6418 w6434] -> w6368
                      tunnel: [w6419 w6433] -> w6367
                      tunnel: [w6415 sgl 1.0 ("millisecond timer value")] -> w6375
                      tunnel: w6327 -> [w6416 _]
                      tunnel: w6366 -> [w6414 w6430]
                      tunnel: [w6414 w6431] -> w6365
                      tunnel: w6361 -> [w6413 w6427]
                      tunnel: w6360 -> [w6412 w6425]
                      tunnel: [w6413 w6426] -> w6359
                      tunnel: [w6412 w6424] -> w6358
                      frame False {
                        n3327 = Increment(x=w6416) -> (x+1=w6415:sgl)
                      }
                      frame True {
                        n3328 = local read "Y dim"() -> (w6429:sgl)
                        n3329 = Multiply(x=w6429, y=w6430) -> (x*y=w6422:sgl)
                        n3330 = Multiply(x=w6423, y=u8 0 ("millisecond timer value")) -> (x*y=w6433:u8[][])
                        n3331 = Multiply(x=u8 0 ("millisecond timer value"), y=w6436) -> (x*y=w6435:u32[][])
                        n3332 = Increment(x=w6430) -> (x+1=w6431:sgl)
                        n3333 = Replace Array Subset(array=w6427, new element=w6428, index (row)=0 ("disabled index (row)"), index (col)=w6422) -> (w6426:u8[][])
                        n3334 = Replace Array Subset(array=w6425, new element=w6423, index (row)=0 ("disabled index (row)"), index (col)=w6422) -> (w6424:u8[][])
                        n3335 = Multiply(x=w6428, y=u8 0 ("millisecond timer value")) -> (x*y=w6434:u8[][])
                      }
                    }
                    n3336 = Round Toward +Infinity(x=w6326) -> (ceil(x): smallest int >= x=w6325:sgl)
                    "#" <- w6325
                    n3337 = Unbundle By Name(w6395) -> ("status"=w6393:bool)
                    n3338 = Tick Count (ms)() -> (millisecond timer value=w6385:u32)
                    n3339 = Unbundle By Name(w6377) -> ("status"=w6379:bool)
                    n3340 = Unbundle By Name(w6394) -> ("status"=w6392:bool)
                    n3341 = local read "stop 2"() -> (w6397:bool)
                    n3342 = local read "End experiment"() -> (w6389:bool)
                    n3343 = Compound Arithmetic op=OR(w6397, w6396, w6393, w6392, w6391, w6379, w6370, w6371, w6389) -> (w6390:bool)
                    "#" <- w6327
                  }
                  n3344 = Decrement(x=w6280) -> (x-1=w6281:sgl)
                }
